vi "Emballage_BDD_scann_portcom.vi"(8 "error in (no error)":errorcluster) -> (0 "Error out":errorcluster)   [LabVIEW 2020]
panel:
  in  "btn_defaut":bool
  in  "stop":bool
  in  "Btn_RechercherPortComScanner":bool
  out "Port Com":refnum<visa-resource-name>
  in  "Famille":u16(ring) items=["Autre", "FLATPROP", "S0020002", "S1121229", "S1121289", "S1121437", "S1220096", "S0020010", "S1121066", "S1220009", "S1121065", "F011106", "F011107", "S1210017", "FASPROP", "CHIPPROP_2W", "CHIPPROP_3W", "NoTest", "CHIPREG"]
  # "Veuillez sélectionner une famille pour recherche \nle port com du lecteur de code barre correspondant\nCliquer sur défaut pour mettre par défaut."
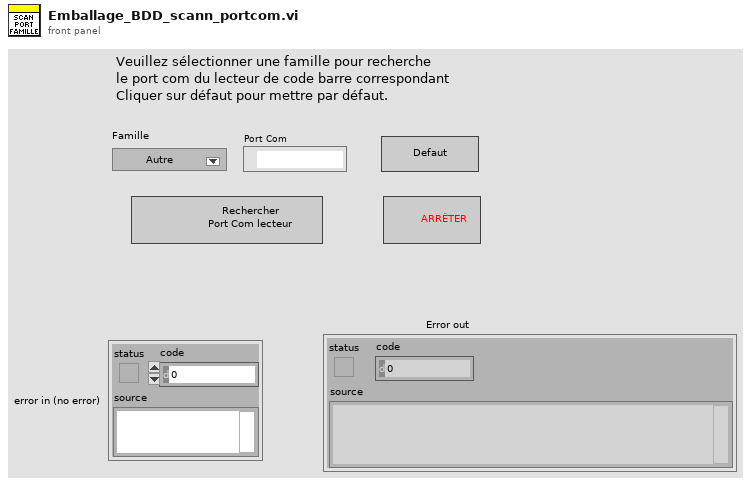
[diagram p1: front panel]
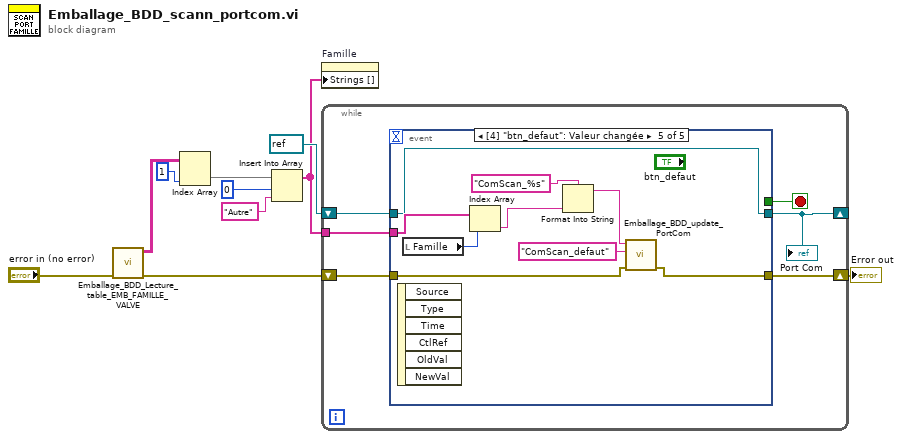
[diagram p0: block diagram]
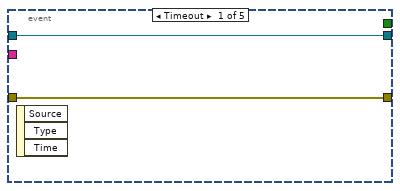
[diagram p2: hidden frame]
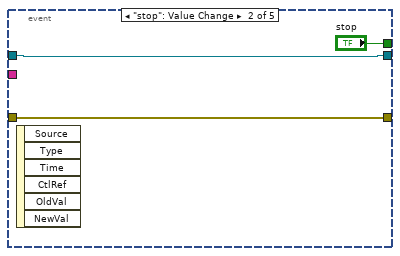
[diagram p3: hidden frame]
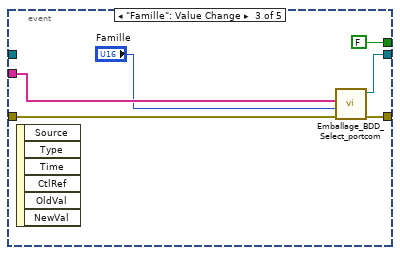
[diagram p4: hidden frame]
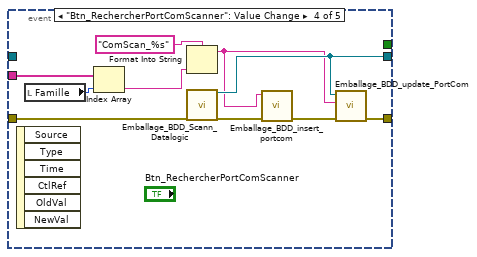
[diagram p5: hidden frame]
diagram:
  n1 = call "Emballage_BDD_Lecture_table_EMB_FAMILLE_VALVE.vi"("entrée d'erreur (pas d'erreur)"="error in (no error)") -> ("sortie d'erreur"=w7:errorcluster, "données"=w8:string[][])  [unwired: 9 in]
  n2 = Index Array(array=w8, index (col)=1 ("indice désactivé (col)")) -> (element=w4:string[])  [unwired: 1 in]
  n3 = Insert Into Array(array=w4, index=0 ("indice"), new element="Autre" ("nouvel élément/sous-tableau")) -> (w1:string[])
  n4 = property on="Famille" class="MDér (strict)"("Strings []"=w1) -> ()  [unwired: 2 in, 2 out]
  n5 = while {
    shift-right: [w15] -> w6
    shift-left: w7 -> [w16]
    shift-right: [w11] -> _
    shift-left: refnum<visa-resource-name> refnum ("COM Array") -> [w13]
    tunnel: w1 -> [w12]
    stop <- w14 stop-if-true
    n6 = event shown="[4] \"btn_defaut\": Valeur changée" {
      selector: _ -> [_ _ _ _ _]
      dyn-events: _ -> [_ _ _ _ _]
      timeout: _ -> [_ _ _ _ _]
      tunnel: w16 -> [w18 w20 w27 w37 w45]
      tunnel: w12 -> [_ _ w26 w33 w41]
      tunnel: [w18 w20 w25 w36 w44] -> w15
      tunnel: [w17 w19 w24 w35 w38] -> w11
      tunnel: [_ "stop" FALSE ("stop") _ _] -> w14
      tunnel: w13 -> [w17 w19 _ _ w38]
      event Timeout {
        n7 = event-data() -> ()  [unwired: 1 in, 3 out]
      }
      event "stop": Value Change {
        n8 = event-data() -> ()  [unwired: 1 in, 6 out]
      }
      event "Famille": Value Change {
        n9 = event-data() -> ()  [unwired: 1 in, 6 out]
        n10 = call "Emballage_BDD_Select_portcom.vi"("entrée d'erreur (pas d'erreur)"=w27, "Famille"="Famille", "Familles"=w26) -> ("sortie d'erreur"=w25:errorcluster, "Refnum VISA en sortie"=w24:refnum<visa-resource-name>)  [unwired: 7 in]
      }
      event "Btn_RechercherPortComScanner": Value Change {
        n11 = event-data() -> ()  [unwired: 1 in, 6 out]
        n12 = local read "Famille"() -> (w28:u16)
        n13 = Index Array(array=w33, index=w28) -> (element=w32:string)
        n14 = Format Into String(format string="ComScan_%s" ("champsCom"), w32) -> (resulting string=w29:string)  [unwired: 2 in, 1 out]
        n15 = call "Emballage_BDD_Scann_Datalogic.vi"("error in (no error)"=w37) -> ("COM Array"=w35:refnum<visa-resource-name>, "error out"=w31:errorcluster)  [unwired: 14 in, 3 out]
        n16 = call "Emballage_BDD_insert_portcom.vi"("entrée d'erreur (pas d'erreur)"=w31, "portcom"=w29) -> ("sortie d'erreur"=w30:errorcluster)  [unwired: 9 in]
        n17 = call "Emballage_BDD_update_PortCom.vi"("Error in"=w30, "champsCom"=w29, "PortCom"=w35) -> ("Error out"=w36:errorcluster)  [unwired: 8 in]
      }
      event "btn_defaut": Value Change {
        n18 = event-data() -> ()  [unwired: 1 in, 6 out]
        n19 = local read "Famille"() -> (w39:u16)
        n20 = Index Array(array=w41, index=w39) -> (element=w42:string)
        n21 = Format Into String(format string="ComScan_%s" ("champsCom"), w42) -> (resulting string=w40:string)  [unwired: 2 in, 1 out]
        n22 = call "Emballage_BDD_update_PortCom.vi"("Error in"=w45, "champsCom"="ComScan_defaut", "PortCom"=w40) -> ("Error out"=w44:errorcluster)  [unwired: 8 in]
      }
    }
    "Port Com" <- w11
  }
  "Error out" <- w6
